vi "niFpgaIPINodeRegularExpressions.vi"() -> ()   [LabVIEW 2017]
panel:
  in  "GenericTypeRegex":string="^\\b(constant|variable|signal|file|termianl|quantity)\\b"
  in  "PortModeRegex":string="^\\b(in|out|inout|buffer|linkage)\\b"
  in  "EntityRegexTemplate":string="ENTITY[\\s\\t\\n\\r\\f\\v]*ENTITY_NAME[\\s\\t\\n\\r\\f\\v]*IS[\\s\\t\\n\\r\\f\\v]*.*?[\\s\\t\\n\\r\\f\\v]*(BEGIN[\\s\\t\\n\\r\\f\\v]*.*)?[\\s\\t\\n\\r\\f\\v]*END[\\s\\t\\n\\r\\f\\v]*(ENTITY)?[\\s\\t\\n\\r\\f\\v]*ENTITY_NAME[\\s\\t\\n\\r\\f\\v]*;"
  in  "EntityDeclarationRegex":string="ENTITY[\\s\\t\\n\\r\\f\\v]*([a-zA-Z]([_a-zA-Z0-9])*|\\\\([[\\s\\t\\n\\r\\f\\v]*a-zA-Z0-9&'\\(\\)\\+,-\\./:;<=>\\|\\\\#\\[\\]_!\\$%@\\?\\^`\\{\\}~])+\\\\)[\\s\\t\\n\\r\\f\\v]*IS[\\s\\t\\n\\r\\f\\v]*.*?[\\s\\t\\n\\r\\f\\v]*(BEGIN[\\s\\t\\n\\r\\f\\v]*.*)?[\\s\\t\\n\\r\\f\\v]*END[\\s\\t\\n\\r\\f\\v]*(ENTITY)?[\\s\\t\\n\\r\\f\\v]*(([a-zA-Z]([_a-zA-Z0-9])*|\\\\([[\\s\\t\\n\\r\\f\\v]*a-zA-Z0-9&'\\(\\)\\+,-\\./:;<=>\\|\\\\#\\[\\]_!\\$%@\\?\\^`\\{\\}~])+\\\\))?[\\s\\t\\n\\r\\f\\v]*;"
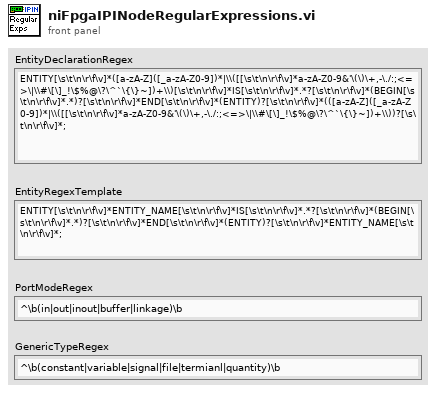
[diagram p1: front panel]
diagram:
